vi "test_read-nmea-data2.vi"() -> ()   [LabVIEW 2019] (continued)
,4.469,K,A*2E\n\t\n15:14:32.27\tF9P\t$GNGGA,061434.00,3723.60300,N,12656.97670,E,1,12,0.66,44.3,M,18.5,M,,*73\n\t\n15:14:32.29\tF9P\t$GNGSA,A,3,12,06,19,05,17,09,04,02,,,,,1.17,0.66,0.97,1*09\n\t\n15:14:32.31\tF9P\t$GNGSA,A,3,85,70,71,84,,,,,,,,,1.17,0.66,0.97,2*0B\n\t\n15:14:32.33\tF9P\t$GNGSA,A,3,36,19,11,04,09,12,,,,,,,1.17,0.66,0.97,3*09\n\t\n15:14:32.35\tF9P\t$GNGSA,A,3,14,11,33,,,,,,,,,,1.17,0.66,0.97,4*08\n\t\n15:14:32.37\tF9P\t$GPGSV,3,1,09,02,55,320,29,04,17,043,28,05,38,248,28,06,64,050,31,1*61\n\t\n15:14:32.39\tF9P\t$GPGSV,3,2,09,09,44,073,25,12,23,276,30,17,32,154,27,19,51,157,44,1*69\n\t\n15:14:32.41\tF9P\t$GPGSV,3,3,09,25,12,306,20,1*5E\n\t\n15:14:32.43\tF9P\t$GPGSV,3,1,09,02,55,320,,04,17,043,25,05,38,248,18,06,64,050,25,6*66\n\t\n15:14:32.45\tF9P\t$GPGSV,3,2,09,09,44,073,26,12,23,276,13,17,32,154,20,19,51,157,,6*6B\n\t\n15:14:32.47\tF9P\t$GPGSV,3,3,09,25,12,306,,6*5B\n\t\n15:14:32.49\tF9P\t$GLGSV,2,1,08,69,10,031,27,70,70,037,22,71,54,207,27,72,05,210,,1*7A\n\t\n15:14:32.51\tF9P\t$GLGSV,2,2,08,77,01,324,,84,19,123,19,85,70,070,32,86,37,330,,1*7E\n\t\n15:14:32.53\tF9P\t$GLGSV,2,1,08,69,10,031,22,70,70,037,,71,54,207,30,72,05,210,,3*7B\n\t\n15:14:32.55\tF9P\t$GLGSV,2,2,08,77,01,324,,84,19,123,21,85,70,070,25,86,37,330,,3*71\n\t\n15:14:32.57\tF9P\t$GAGSV,2,1,08,02,08,296,12,04,67,115,29,09,33,193,24,11,72,001,25,7*70\n\t\n15:14:32.59\tF9P\t$GAGSV,2,2,08,12,39,103,30,19,25,045,23,25,08,248,,36,27,309,19,7*7F\n\t\n15:14:32.61\tF9P\t$GAGSV,2,1,08,02,08,296,,04,67,115,,09,33,193,,11,72,001,,2*7C\n\t\n15:14:32.63\tF9P\t$GAGSV,2,2,08,12,39,103,,19,25,045,,25,08,248,,36,27,309,,2*70\n\t\n15:14:32.65\tF9P\t$GBGSV,2,1,06,07,,,28,11,48,133,39,14,87,101,26,28,,,24,1*7B\n\t\n15:14:32.67\tF9P\t$GBGSV,2,2,06,33,62,220,34,34,,,38,1*4F\n\t\n15:14:32.69\tF9P\t$GBGSV,1,1,03,11,48,133,29,14,87,101,27,33,62,220,,3*4A\n\t\n15:14:32.71\tF9P\t$GNGLL,3723.60300,N,12656.97670,E,061434.00,A,A*7A\n\t\n15:14:32.73\tF9P\t\t\n15:14:32.75\tF9P\t\t\n15:14:32.77\tF9P\t\t\n15:14:32.79\tF9P\t\t\n15:14:32.81\tF9P\t\t\n15:14:32.83\tF9P\t\t\n15:14:32.85\tF9P\t\t\n15:14:32.87\tF9P\t\t\n15:14:32.89\tF9P\t\t\n15:14:32.91\tF9P\t\t\n15:14:32.93\tF9P\t\t\n15:14:32.95\tF9P\t\t\n15:14:32.97\tF9P\t\t\n15:14:32.99\tF9P\t\t\n15:14:33.01\tF9P\t\t\n15:14:33.03\tF9P\t\t\n15:14:33.05\tF9P\t\t\n15:14:33.07\tF9P\t\t\n15:14:33.09\tF9P\t\t\n15:14:33.11\tF9P\t\t\n15:14:33.13\tF9P\t\t\n15:14:33.15\tF9P\t\t\n15:14:33.17\tF9P\t\t\n15:14:33.19\tF9P\t\t\n15:14:33.21\tF9P\t\t\n15:14:33.23\tF9P\t$GNRMC,061435.00,A,3723.60368,N,12656.97644,E,1.900,340.64,250720,,,A,V*00\n\t\n15:14:33.25\tF9P\t$GNVTG,340.64,T,,M,1.900,N,3.519,K,A*20\n\t\n15:14:33.27\tF9P\t$GNGGA,061435.00,3723.60368,N,12656.97644,E,1,12,0.66,44.5,M,18.5,M,,*7D\n\t\n15:14:33.29\tF9P\t$GNGSA,A,3,12,06,19,05,17,09,04,02,,,,,1.17,0.66,0.97,1*09\n\t\n15:14:33.31\tF9P\t$GNGSA,A,3,85,70,71,84,,,,,,,,,1.17,0.66,0.97,2*0B\n\t\n15:14:33.33\tF9P\t$GNGSA,A,3,36,19,11,04,09,12,,,,,,,1.17,0.66,0.97,3*09\n\t\n15:14:33.35\tF9P\t$GNGSA,A,3,14,11,33,,,,,,,,,,1.17,0.66,0.97,4*08\n\t\n15:14:33.37\tF9P\t$GPGSV,3,1,09,02,55,320,32,04,17,043,33,05,38,248,21,06,64,050,29,1*61\n\t\n15:14:33.39\tF9P\t$GPGSV,3,2,09,09,44,073,35,12,23,276,23,17,32,154,36,19,51,157,42,1*6C\n\t\n15:14:33.41\tF9P\t$GPGSV,3,3,09,25,12,306,20,1*5E\n\t\n15:14:33.43\tF9P\t$GPGSV,3,1,09,02,55,320,,04,17,043,24,05,38,248,17,06,64,050,25,6*68\n\t\n15:14:33.45\tF9P\t$GPGSV,3,2,09,09,44,073,31,12,23,276,12,17,32,154,22,19,51,157,,6*6E\n\t\n15:14:33.47\tF9P\t$GPGSV,3,3,09,25,12,306,,6*5B\n\t\n15:14:33.49\tF9P\t$GLGSV,2,1,08,69,10,031,28,70,70,037,22,71,54,207,28,72,05,210,,1*7A\n\t\n15:14:33.51\tF9P\t$GLGSV,2,2,08,77,01,324,,84,19,123,19,85,70,070,33,86,37,330,,1*7F\n\t\n15:14:33.53\tF9P\t$GLGSV,2,1,08,69,10,031,21,70,70,037,,71,54,207,22,72,05,210,,3*7B\n\t\n15:14:33.55\tF9P\t$GLGSV,2,2,08,77,01,324,,84,19,123,21,85,70,070,24,86,37,330,,3*70\n\t\n15:14:33.57\tF9P\t$GAGSV,2,1,08,02,08,296,12,04,67,115,34,09,33,193,29,11,72,001,26,7*72\n\t\n15:14:33.59\tF9P\t$GAGSV,2,2,08,12,39,103,31,19,25,045,29,25,08,248,,36,27,309,18,7*75\n\t\n15:14:33.61\tF9P\t$GAGSV,2,1,08,02,08,296,,04,67,115,,09,33,193,,11,72,001,,2*7C\n\t\n15:14:33.63\tF9P\t$GAGSV,2,2,08,12,39,103,,19,25,045,,25,08,248,,36,27,309,,2*70\n\t\n15:14:33.65\tF9P\t$GBGSV,2,1,06,07,,,28,11,48,133,32,14,87,101,27,28,,,35,1*71\n\t\n15:14:33.67\tF9P\t$GBGSV,2,2,06,33,62,220,25,34,,,37,1*40\n\t\n15:14:33.69\tF9P\t$GBGSV,1,1,03,11,48,133,,14,87,101,26,33,62,220,,3*40\n\t\n15:14:33.71\tF9P\t$GNGLL,3723.60368,N,12656.97644,E,061435.00,A,A*72\n\t\n15:14:33.73\tF9P\t\t\n15:14:33.75\tF9P\t\t\n15:14:33.77\tF9P\t\t\n15:14:33.79\tF9P\t\t\n15:14:33.81\tF9P\t\t\n15:14:33.83\tF9P\t\t\n15:14:33.85\tF9P\t\t\n15:14:33.87\tF9P\t\t\n15:14:33.89\tF9P\t\t\n15:14:33.91\tF9P\t\t\n15:14:33.93\tF9P\t\t\n15:14:33.95\tF9P\t\t\n15:14:33.97\tF9P\t\t\n15:14:33.99\tF9P\t\t\n15:14:34.01\tF9P\t\t\n15:14:34.03\tF9P\t\t\n15:14:34.05\tF9P\t\t\n15:14:34.07\tF9P\t\t\n15:14:34.09\tF9P\t\t\n15:14:34.11\tF9P\t\t\n15:14:34.13\tF9P\t\t\n15:14:34.15\tF9P\t\t\n15:14:34.17\tF9P\t\t\n15:14:34.19\tF9P\t\t\n15:14:34.21\tF9P\t\t\n15:14:34.23\tF9P\t$GNRMC,061436.00,A,3723.60422,N,12656.97608,E,1.540,329.07,250720,,,A,V*00\n\t\n15:14:34.25\tF9P\t$GNVTG,329.07,T,,M,1.540,N,2.852,K,A*21\n\t\n15:14:34.27\tF9P\t$GNGGA,061436.00,3723.60422,N,12656.97608,E,1,12,0.66,44.8,M,18.5,M,,*72\n\t\n15:14:34.29\tF9P\t$GNGSA,A,3,12,06,19,05,17,09,04,02,,,,,1.17,0.66,0.97,1*09\n\t\n15:14:34.31\tF9P\t$GNGSA,A,3,85,70,71,84,,,,,,,,,1.17,0.66,0.97,2*0B\n\t\n15:14:34.33\tF9P\t$GNGSA,A,3,36,19,11,04,09,12,,,,,,,1.17,0.66,0.97,3*09\n\t\n15:14:34.35\tF9P\t$GNGSA,A,3,14,11,33,,,,,,,,,,1.17,0.66,0.97,4*08\n\t\n15:14:34.37\tF9P\t$GPGSV,3,1,09,02,55,320,30,04,17,043,32,05,38,248,25,06,64,050,33,1*6D\n\t\n15:14:34.39\tF9P\t$GPGSV,3,2,09,09,44,073,36,12,23,276,23,17,32,154,33,19,51,157,38,1*67\n\t\n15:14:34.41\tF9P\t$GPGSV,3,3,09,25,12,306,18,1*55\n\t\n15:14:34.43\tF9P\t$GPGSV,3,1,09,02,55,320,,04,17,043,23,05,38,248,17,06,64,050,24,6*6E\n\t\n15:14:34.45\tF9P\t$GPGSV,3,2,09,09,44,073,24,12,23,276,12,17,32,154,30,19,51,157,,6*69\n\t\n15:14:34.47\tF9P\t$GPGSV,3,3,09,25,12,306,,6*5B\n\t\n15:14:34.49\tF9P\t$GLGSV,2,1,08,69,10,031,30,70,70,037,23,71,54,207,33,72,05,210,,1*78\n\t\n15:14:34.51\tF9P\t$GLGSV,2,2,08,77,01,324,,84,19,123,21,85,70,070,28,86,37,330,,1*7E\n\t\n15:14:34.53\tF9P\t$GLGSV,2,1,08,69,10,031,21,70,70,037,,71,54,207,22,72,05,210,,3*7B\n\t\n15:14:34.55\tF9P\t$GLGSV,2,2,08,77,01,324,,84,19,123,29,85,70,070,23,86,37,330,,3*7F\n\t\n15:14:34.57\tF9P\t$GAGSV,2,1,08,02,08,296,10,04,67,115,31,09,33,193,29,11,72,001,25,7*76\n\t\n15:14:34.59\tF9P\t$GAGSV,2,2,08,12,39,103,32,19,25,045,22,25,08,248,,36,27,309,19,7*7C\n\t\n15:14:34.61\tF9P\t$GAGSV,2,1,08,02,08,296,,04,67,115,,09,33,193,,11,72,001,,2*7C\n\t\n15:14:34.63\tF9P\t$GAGSV,2,2,08,12,39,103,,19,25,045,,25,08,248,,36,27,309,,2*70\n\t\n15:14:34.65\tF9P\t$GBGSV,2,1,06,07,,,29,11,48,133,37,14,87,101,27,28,,,34,1*74\n\t\n15:14:34.67\tF9P\t$GBGSV,2,2,06,33,62,220,31,34,,,39,1*4B\n\t\n15:14:34.69\tF9P\t$GBGSV,1,1,03,11,48,133,29,14,87,101,26,33,62,220,,3*4B\n\t\n15:14:34.71\tF9P\t$GNGLL,3723.60422,N,12656.97608,E,061436.00,A,A*70\n\t\n15:14:34.73\tF9P\t\t\n15:14:34.75\tF9P\t\t\n15:14:34.77\tF9P\t\t\n15:14:34.79\tF9P\t\t\n15:14:34.81\tF9P\t\t\n15:14:34.83\tF9P\t\t\n15:14:34.85\tF9P\t\t\n15:14:34.87\tF9P\t\t\n15:14:34.89\tF9P\t\t\n15:14:34.91\tF9P\t\t\n15:14:34.93\tF9P\t\t\n15:14:34.95\tF9P\t\t\n15:14:34.97\tF9P\t\t\n15:14:34.99\tF9P\t\t\n15:14:35.01\tF9P\t\t\n15:14:35.03\tF9P\t\t\n15:14:35.05\tF9P\t\t\n15:14:35.07\tF9P\t\t\n15:14:35.09\tF9P\t\t\n15:14:35.11\tF9P\t\t\n15:14:35.13\tF9P\t\t\n15:14:35.15\tF9P\t\t\n15:14:35.17\tF9P\t\t\n15:14:35.19\tF9P\t\t\n15:14:35.21\tF9P\t\t\n15:14:35.23\tF9P\t$GNRMC,061437.00,A,3723.60450,N,12656.97555,E,1.519,295.19,250720,,,A,V*0A\n\t\n15:14:35.25\tF9P\t$GNVTG,295.19,T,,M,1.519,N,2.812,K,A*20\n\t\n15:14:35.27\tF9P\t$GNGGA,061437.00,3723.60450,N,12656.97555,E,1,12,0.66,45.5,M,18.5,M,,*71\n\t\n15:14:35.29\tF9P\t$GNGSA,A,3,12,06,19,05,17,09,04,02,,,,,1.17,0.66,0.97,1*09\n\t\n15:14:35.31\tF9P\t$GNGSA,A,3,85,70,71,84,,,,,,,,,1.17,0.66,0.97,2*0B\n\t\n15:14:35.33\tF9P\t$GNGSA,A,3,36,19,11,04,09,12,,,,,,,1.17,0.66,0.97,3*09\n\t\n15:14:35.35\tF9P\t$GNGSA,A,3,14,11,33,,,,,,,,,,1.17,0.66,0.97,4*08\n\t\n15:14:35.37\tF9P\t$GPGSV,3,1,09,02,55,320,30,04,17,043,33,05,38,248,26,06,64,050,31,1*6D\n\t\n15:14:35.39\tF9P\t$GPGSV,3,2,09,09,44,073,38,12,23,276,23,17,32,154,41,19,51,157,31,1*65\n\t\n15:14:35.41\tF9P\t$GPGSV,3,3,09,25,12,306,17,1*5A\n\t\n15:14:35.43\tF9P\t$GPGSV,3,1,09,02,55,320,,04,17,043,24,05,38,248,17,06,64,050,25,6*68\n\t\n15:14:35.45\tF9P\t$GPGSV,3,2,09,09,44,073,24,12,23,276,11,17,32,154,21,19,51,157,,6*6A\n\t\n15:14:35.47\tF9P\t$GPGSV,3,3,09,25,12,306,,6*5B\n\t\n15:14:35.49\tF9P\t$GLGSV,2,1,08,69,10,031,28,70,70,037,23,71,54,207,30,72,05,210,,1*72\n\t\n15:14:35.51\tF9P\t$GLGSV,2,2,08,77,01,324,,84,19,123,22,85,70,070,33,86,37,330,,1*77\n\t\n15:14:35.53\tF9P\t$GLGSV,2,1,08,69,10,031,20,70,70,037,,71,54,207,21,72,05,210,,3*79\n\t\n15:14:35.55\tF9P\t$GLGSV,2,2,08,77,01,324,,84,19,123,29,85,70,070,22,86,37,330,,3*7E\n\t\n15:14:35.57\tF9P\t$GAGSV,2,1,08,02,08,296,10,04,67,115,36,09,33,193,28,11,72,001,24,7*71\n\t\n15:14:35.59\tF9P\t$GAGSV,2,2,08,12,39,103,33,19,25,045,29,25,08,248,,36,27,309,18,7*77\n\t\n15:14:35.61\tF9P\t$GAGSV,2,1,08,02,08,296,,04,67,115,,09,33,193,,11,72,001,,2*7C\n\t\n15:14:35.63\tF9P\t$GAGSV,2,2,08,12,39,103,,19,25,045,,25,08,248,,36,27,309,,2*70\n\t\n15:14:35.65\tF9P\t$GBGSV,2,1,06,07,,,30,11,48,133,35,14,87,101,27,28,,,31,1*7B\n\t\n15:14:35.67\tF9P\t$GBGSV,2,2,06,33,62,220,30,34,,,37,1*44\n\t\n15:14:35.69\tF9P\t$GBGSV,1,1,03,11,48,133,30,14,87,101,31,33,62,220,,3*45\n\t\n15:14:35.71\tF9P\t$GNGLL,3723.60450,N,12656.97555,E,061437.00,A,A*7F\n\t\n15:14:35.73\tF9P\t\t\n15:14:35.75\tF9P\t\t\n15:14:35.77\tF9P\t\t\n15:14:35.79\tF9P\t\t\n15:14:35.81\tF9P\t\t\n15:14:35.83\tF9P\t\t\n15:14:35.85\tF9P\t\t\n15:14:35.87\tF9P\t\t\n15:14:35.89\tF9P\t\t\n15:14:35.91\tF9P\t\t\n15:14:35.93\tF9P\t\t\n15:14:35.95\tF9P\t\t\n15:14:35.97\tF9P\t\t\n15:14:35.99\tF9P\t\t\n15:14:36.01\tF9P\t\t\n15:14:36.03\tF9P\t\t\n15:14:36.05\tF9P\t\t\n15:14:36.07\tF9P\t\t\n15:14:36.09\tF9P\t\t\n15:14:36.11\tF9P\t\t\n15:14:36.13\tF9P\t\t\n15:14:36.15\tF9P\t\t\n15:14:36.17\tF9P\t\t\n15:14:36.19\tF9P\t\t\n15:14:36.21\tF9P\t\t\n15:14:36.23\tF9P\t$GNRMC,061438.00,A,3723.60462,N,12656.97495,E,1.927,273.84,250720,,,A,V*04\n\t\n15:14:36.25\tF9P\t$GNVTG,273.84,T,,M,1.927,N,3.569,K,A*2D\n\t\n15:14:36.27\tF9P\t$GNGGA,061438.00,3723.60462,N,12656.97495,E,1,12,0.64,45.4,M,18.5,M,,*71\n\t\n15:14:36.29\tF9P\t$GNGSA,A,3,12,06,19,05,17,09,04,02,,,,,1.17,0.64,0.97,1*0B\n\t\n15:14:36.31\tF9P\t$GNGSA,A,3,85,70,71,84,,,,,,,,,1.17,0.64,0.97,2*09\n\t\n15:14:36.33\tF9P\t$GNGSA,A,3,36,19,11,04,09,12,,,,,,,1.17,0.64,0.97,3*0B\n\t\n15:14:36.35\tF9P\t$GNGSA,A,3,14,11,33,,,,,,,,,,1.17,0.64,0.97,4*0A\n\t\n15:14:36.37\tF9P\t$GPGSV,3,1,09,02,55,320,27,04,17,043,39,05,38,248,32,06,64,050,25,1*61\n\t\n15:14:36.39\tF9P\t$GPGSV,3,2,09,09,44,073,39,12,23,276,23,17,32,154,29,19,51,157,31,1*6A\n\t\n15:14:36.41\tF9P\t$GPGSV,3,3,09,25,12,306,16,1*5B\n\t\n15:14:36.43\tF9P\t$GPGSV,3,1,09,02,55,320,,04,17,043,27,05,38,248,20,06,64,050,31,6*6A\n\t\n15:14:36.45\tF9P\t$GPGSV,3,2,09,09,44,073,31,12,23,276,11,17,32,154,22,19,51,157,,6*6D\n\t\n15:14:36.47\tF9P\t$GPGSV,3,3,09,25,12,306,,6*5B\n\t\n15:14:36.49\tF9P\t$GLGSV,2,1,08,69,10,031,27,70,70,037,32,71,54,207,30,72,05,210,,1*7D\n\t\n15:14:36.51\tF9P\t$GLGSV,2,2,08,77,01,324,,84,19,123,23,85,70,070,40,86,37,330,,1*72\n\t\n15:14:36.53\tF9P\t$GLGSV,2,1,08,69,10,031,19,70,70,037,,71,54,207,19,72,05,210,,3*78\n\t\n15:14:36.55\tF9P\t$GLGSV,2,2,08,77,01,324,,84,19,123,29,85,70,070,22,86,37,330,,3*7E\n\t\n15:14:36.57\tF9P\t$GAGSV,2,1,08,02,08,296,09,04,67,115,37,09,33,193,28,11,72,001,25,7*79\n\t\n15:14:36.59\tF9P\t$GAGSV,2,2,08,12,39,103,30,19,25,045,21,25,08,248,,36,27,309,18,7*7C\n\t\n15:14:36.61\tF9P\t$GAGSV,2,1,08,02,08,296,,04,67,115,,09,33,193,,11,72,001,,2*7C\n\t\n15:14:36.63\tF9P\t$GAGSV,2,2,08,12,39,103,,19,25,045,,25,08,248,,36,27,309,,2*70\n\t\n15:14:36.65\tF9P\t$GBGSV,2,1,06,07,,,29,11,48,133,37,14,87,101,31,28,,,26,1*70\n\t\n15:14:36.67\tF9P\t$GBGSV,2,2,06,33,62,220,24,34,,,39,1*4F\n\t\n15:14:36.69\tF9P\t$GBGSV,1,1,03,11,48,133,,14,87,101,25,33,62,220,,3*43\n\t\n15:14:36.71\tF9P\t$GNGLL,3723.60462,N,12656.97495,E,061438.00,A,A*7C\n\t\n15:14:36.73\tF9P\t\t\n15:14:36.75\tF9P\t\t\n15:14:36.77\tF9P\t\t\n15:14:36.79\tF9P\t\t\n15:14:36.81\tF9P\t\t\n15:14:36.83\tF9P\t\t\n15:14:36.85\tF9P\t\t\n15:14:36.87\tF9P\t\t\n15:14:36.89\tF9P\t\t\n15:14:36.91\tF9P\t\t\n15:14:36.93\tF9P\t\t\n15:14:36.95\tF9P\t\t\n15:14:36.97\tF9P\t\t\n15:14:36.99\tF9P\t\t\n15:14:37.01\tF9P\t\t\n15:14:37.03\tF9P\t\t\n15:14:37.05\tF9P\t\t\n15:14:37.07\tF9P\t\t\n15:14:37.09\tF9P\t\t\n15:14:37.11\tF9P\t\t\n15:14:37.13\tF9P\t\t\n15:14:37.15\tF9P\t\t\n15:14:37.17\tF9P\t\t\n15:14:37.19\tF9P\t\t\n15:14:37.21\tF9P\t\t\n15:14:37.23\tF9P\t$GNRMC,061439.00,A,3723.60479,N,12656.97386,E,3.046,263.46,250720,,,A,V*09\n\t\n15:14:37.25\tF9P\t$GNVTG,263.46,T,,M,3.046,N,5.641,K,A*21\n\t\n15:14:37.27\tF9P\t$GNGGA,061439.00,3723.60479,N,12656.97386,E,1,12,0.66,45.2,M,18.5,M,,*7B\n\t\n15:14:37.29\tF9P\t$GNGSA,A,3,12,06,19,05,17,09,04,02,,,,,1.17,0.66,0.97,1*09\n\t\n15:14:37.31\tF9P\t$GNGSA,A,3,85,70,71,84,,,,,,,,,1.17,0.66,0.97,2*0B\n\t\n15:14:37.33\tF9P\t$GNGSA,A,3,36,19,11,04,09,12,,,,,,,1.17,0.66,0.97,3*09\n\t\n15:14:37.35\tF9P\t$GNGSA,A,3,14,11,33,,,,,,,,,,1.17,0.66,0.97,4*08\n\t\n15:14:37.37\tF9P\t$GPGSV,3,1,09,02,55,320,28,04,17,043,27,05,38,248,32,06,64,050,30,1*65\n\t\n15:14:37.39\tF9P\t$GPGSV,3,2,09,09,44,073,41,12,23,276,23,17,32,154,37,19,51,157,34,1*6F\n\t\n15:14:37.41\tF9P\t$GPGSV,3,3,09,25,12,306,12,1*5F\n\t\n15:14:37.43\tF9P\t$GPGSV,3,1,09,02,55,320,,04,17,043,31,05,38,248,27,06,64,050,22,6*68\n\t\n15:14:37.45\tF9P\t$GPGSV,3,2,09,09,44,073,30,12,23,276,13,17,32,154,21,19,51,157,,6*6D\n\t\n15:14:37.47\tF9P\t$GPGSV,3,3,09,25,12,306,,6*5B\n\t\n15:14:37.49\tF9P\t$GLGSV,2,1,08,69,10,031,26,70,70,037,26,71,54,207,34,72,05,210,,1*7D\n\t\n15:14:37.51\tF9P\t$GLGSV,2,2,08,77,01,324,,84,19,123,21,85,70,070,30,86,37,330,,1*77\n\t\n15:14:37.53\tF9P\t$GLGSV,2,1,08,69,10,031,17,70,70,037,,71,54,207,20,72,05,210,,3*7C\n\t\n15:14:37.55\tF9P\t$GLGSV,2,2,08,77,01,324,,84,19,123,30,85,70,070,22,86,37,330,,3*76\n\t\n15:14:37.57\tF9P\t$GAGSV,2,1,08,02,08,296,10,04,67,115,31,09,33,193,21,11,72,001,24,7*7F\n\t\n15:14:37.59\tF9P\t$GAGSV,2,2,08,12,39,103,30,19,25,045,34,25,08,248,,36,27,309,19,7*79\n\t\n15:14:37.61\tF9P\t$GAGSV,2,1,08,02,08,296,,04,67,115,,09,33,193,,11,72,001,,2*7C\n\t\n15:14:37.63\tF9P\t$GAGSV,2,2,08,12,39,103,,19,25,045,,25,08,248,,36,27,309,,2*70\n\t\n15:14:37.65\tF9P\t$GBGSV,2,1,06,07,,,20,11,48,133,39,14,87,101,25,28,,,34,1*71\n\t\n15:14:37.67\tF9P\t$GBGSV,2,2,06,33,62,220,31,34,,,37,1*45\n\t\n15:14:37.69\tF9P\t$GBGSV,1,1,03,11,48,133,,14,87,101,,33,62,220,,3*44\n\t\n15:14:37.71\tF9P\t$GNGLL,3723.60479,N,12656.97386,E,061439.00,A,A*72\n\t\n15:14:37.73\tF9P\t\t\n15:14:37.75\tF9P\t\t\n15:14:37.77\tF9P\t\t\n15:14:37.79\tF9P\t\t\n15:14:37.81\tF9P\t\t\n15:14:37.83\tF9P\t\t\n15:14:37.85\tF9P\t\t\n15:14:37.87\tF9P\t\t\n15:14:37.89\tF9P\t\t\n15:14:37.91\tF9P\t\t\n15:14:37.93\tF9P\t\t\n15:14:37.95\tF9P\t\t\n15:14:37.97\tF9P\t\t\n15:14:37.99\tF9P\t\t\n15:14:38.01\tF9P\t\t\n15:14:38.03\tF9P\t\t\n15:14:38.05\tF9P\t\t\n15:14:38.07\tF9P\t\t\n15:14:38.09\tF9P\t\t\n15:14:38.11\tF9P\t\t\n15:14:38.13\tF9P\t\t\n15:14:38.15\tF9P\t\t\n15:14:38.17\tF9P\t\t\n15:14:38.19\tF9P\t\t\n15:14:38.21\tF9P\t\t\n15:14:38.23\tF9P\t$GNRMC,061440.00,A,3723.60491,N,12656.97306,E,2.486,257.81,250720,,,A,V*0C\n\t\n15:14:38.25\tF9P\t$GNVTG,257.81,T,,M,2.486,N,4.605,K,A*25\n\t\n15:14:38.27\tF9P\t$GNGGA,061440.00,3723.60491,N,12656.97306,E,1,12,0.63,44.8,M,18.5,M,,*75\n\t\n15:14:38.29\tF9P\t$GNGSA,A,3,12,06,19,05,17,09,04,02,,,,,1.14,0.63,0.95,1*0D\n\t\n15:14:38.31\tF9P\t$GNGSA,A,3,85,70,71,84,,,,,,,,,1.14,0.63,0.95,2*0F\n\t\n15:14:38.33\tF9P\t$GNGSA,A,3,36,19,11,04,09,12,,,,,,,1.14,0.63,0.95,3*0D\n\t\n15:14:38.35\tF9P\t$GNGSA,A,3,14,11,33,,,,,,,,,,1.14,0.63,0.95,4*0C\n\t\n15:14:38.37\tF9P\t$GPGSV,3,1,09,02,55,320,28,04,17,043,41,05,38,248,34,06,64,050,31,1*62\n\t\n15:14:38.39\tF9P\t$GPGSV,3,2,09,09,44,073,34,12,23,276,23,17,32,154,35,19,51,157,35,1*6E\n\t\n15:14:38.41\tF9P\t$GPGSV,3,3,09,25,12,306,10,1*5D\n\t\n15:14:38.43\tF9P\t$GPGSV,3,1,09,02,55,320,,04,17,043,25,05,38,248,26,06,64,050,25,6*6B\n\t\n15:14:38.45\tF9P\t$GPGSV,3,2,09,09,44,073,29,12,23,276,15,17,32,154,20,19,51,157,,6*62\n\t\n15:14:38.47\tF9P\t$GPGSV,3,3,09,25,12,306,,6*5B\n\t\n15:14:38.49\tF9P\t$GLGSV,2,1,08,69,10,031,27,70,70,037,25,71,54,207,36,72,05,210,,1*7D\n\t\n15:14:38.51\tF9P\t$GLGSV,2,2,08,77,01,324,,84,19,123,22,85,69,072,32,86,37,330,,1*7C\n\t\n15:14:38.53\tF9P\t$GLGSV,2,1,08,69,10,031,20,70,70,037,,71,54,207,24,72,05,210,,3*7C\n\t\n15:14:38.55\tF9P\t$GLGSV,2,2,08,77,01,324,,84,19,123,25,85,69,072,23,86,37,330,,3*79\n\t\n15:14:38.57\tF9P\t$GAGSV,2,1,08,02,08,296,10,04,67,115,32,09,33,193,33,11,72,001,24,7*7F\n\t\n15:14:38.59\tF9P\t$GAGSV,2,2,08,12,39,103,33,19,25,045,29,25,08,248,,36,27,309,18,7*77\n\t\n15:14:38.61\tF9P\t$GAGSV,2,1,08,02,08,296,,04,67,115,,09,33,193,,11,72,001,,2*7C\n\t\n15:14:38.63\tF9P\t$GAGSV,2,2,08,12,39,103,,19,25,045,,25,08,248,,36,27,309,,2*70\n\t\n15:14:38.65\tF9P\t$GBGSV,2,1,06,07,,,22,11,48,133,33,14,87,101,25,28,,,31,1*7C\n\t\n15:14:38.67\tF9P\t$GBGSV,2,2,06,33,62,220,31,34,,,33,1*41\n\t\n15:14:38.69\tF9P\t$GBGSV,1,1,03,11,48,133,,14,87,101,,33,62,220,,3*44\n\t\n15:14:38.71\tF9P\t$GNGLL,3723.60491,N,12656.97306,E,061440.00,A,A*72\n\t\n15:14:38.73\tF9P\t\t\n15:14:38.75\tF9P\t\t\n15:14:38.77\tF9P\t\t\n15:14:38.79\tF9P\t\t\n15:14:38.81\tF9P\t\t\n15:14:38.83\tF9P\t\t\n15:14:38.85\tF9P\t\t\n15:14:38.87\tF9P\t\t\n15:14:38.89\tF9P\t\t\n15:14:38.91\tF9P\t\t\n15:14:38.93\tF9P\t\t\n15:14:38.95\tF9P\t\t\n15:14:38.97\tF9P\t\t\n15:14:38.99\tF9P\t\t\n15:14:39.01\tF9P\t\t\n15:14:39.03\tF9P\t\t\n15:14:39.05\tF9P\t\t\n15:14:39.07\tF9P\t\t\n15:14:39.09\tF9P\t\t\n15:14:39.11\tF9P\t\t\n15:14:39.13\tF9P\t\t\n15:14:39.15\tF9P\t\t\n15:14:39.17\tF9P\t\t\n15:14:39.19\tF9P\t\t\n15:14:39.21\tF9P\t\t\n15:14:39.23\tF9P\t$GNRMC,061441.00,A,3723.60486,N,12656.97250,E,2.124,246.90,250720,,,A,V*04\n\t\n15:14:39.25\tF9P\t$GNVTG,246.90,T,,M,2.124,N,3.933,K,A*25\n\t\n15:14:39.27\tF9P\t$GNGGA,061441.00,3723.60486,N,12656.97250,E,1,12,0.63,44.9,M,18.5,M,,*71\n\t\n15:14:39.29\tF9P\t$GNGSA,A,3,12,06,19,05,17,09,04,02,,,,,1.14,0.63,0.95,1*0D\n\t\n15:14:39.31\tF9P\t$GNGSA,A,3,85,70,71,84,,,,,,,,,1.14,0.63,0.95,2*0F\n\t\n15:14:39.33\tF9P\t$GNGSA,A,3,36,19,11,04,09,12,,,,,,,1.14,0.63,0.95,3*0D\n\t\n15:14:39.35\tF9P\t$GNGSA,A,3,14,11,33,,,,,,,,,,1.14,0.63,0.95,4*0C\n\t\n15:14:39.37\tF9P\t$GPGSV,3,1,09,02,55,320,31,04,17,043,42,05,38,248,31,06,64,050,33,1*6E\n\t\n15:14:39.39\tF9P\t$GPGSV,3,2,09,09,44,073,38,12,23,276,24,17,32,154,37,19,51,157,32,1*60\n\t\n15:14:39.41\tF9P\t$GPGSV,3,3,09,25,12,306,19,1*54\n\t\n15:14:39.43\tF9P\t$GPGSV,3,1,09,02,55,320,,04,17,043,31,05,38,248,25,06,64,050,25,6*6D\n\t\n15:14:39.45\tF9P\t$GPGSV,3,2,09,09,44,073,30,12,23,276,14,17,32,154,19,19,51,157,,6*61\n\t\n15:14:39.47\tF9P\t$GPGSV,3,3,09,25,12,306,,6*5B\n\t\n15:14:39.49\tF9P\t$GLGSV,2,1,08,69,10,031,27,70,70,037,24,71,54,207,37,72,05,210,,1*7D\n\t\n15:14:39.51\tF9P\t$GLGSV,2,2,08,77,01,324,,84,19,123,21,85,69,072,35,86,38,331,,1*76\n\t\n15:14:39.53\tF9P\t$GLGSV,2,1,08,69,10,031,20,70,70,037,,71,54,207,26,72,05,210,,3*7E\n\t\n15:14:39.55\tF9P\t$GLGSV,2,2,08,77,01,324,,84,19,123,26,85,69,072,23,86,38,331,,3*74\n\t\n15:14:39.57\tF9P\t$GAGSV,2,1,08,02,08,296,08,04,67,115,31,09,33,193,27,11,72,001,23,7*77\n\t\n15:14:39.59\tF9P\t$GAGSV,2,2,08,12,39,103,29,19,25,045,28,25,08,248,,36,27,309,18,7*7D\n\t\n15:14:39.61\tF9P\t$GAGSV,2,1,08,02,08,296,,04,67,115,,09,33,193,,11,72,001,,2*7C\n\t\n15:14:39.63\tF9P\t$GAGSV,2,2,08,12,39,103,,19,25,045,,25,08,248,,36,27,309,,2*70\n\t\n15:14:39.65\tF9P\t$GBGSV,2,1,06,07,,,24,11,48,133,37,14,87,101,25,28,,,26,1*78\n\t\n15:14:39.67\tF9P
